vi "RMS Current Check.vi"(8 "error in":errorcluster, 10 "WaitMoniter Input":T4={"Wait Time(S)"=10.0, "Chamber Temp(Deg C)"=10.0, "Chamber Temp Tolerance(%)"=10.0, "RMS Current(A)"=10.0, "RMS Current Tolerance(%)"=10.0, "Temperature Control"=FALSE, "RMS Control"=FALSE, "RMS Current Min(A)"=10.0, "RMS Current Max(A)"=10.0, "Chamber Temp Min(Deg C)"=10.0, "Chamber Temp Max(Deg C)"=10.0, "HVPPS Current Max(A)"=10.0, "HVPPS Control"=FALSE, "HVPPS Current(A)"=10.0} {"HVPPS Current(A)" format="%#_13g"; "HVPPS Current Max(A)" format="%#_13g"; "Chamber Temp Max(Deg C)" format="%#_13g"; "Chamber Temp Min(Deg C)" format="%#_13g"; "RMS Current Max(A)" format="%#_13g"; "RMS Current Min(A)" format="%#_13g"; "RMS Current Tolerance(%)" format="%#_13g"; "RMS Current(A)" format="%#_13g"; "Chamber Temp Tolerance(%)" format="%#_13g"; "Chamber Temp(Deg C)" format="%#_13g"; "Wait Time(S)" format="%#_13g"}, 11 "Data Cluster":T1={"Chamber Address"={"Starting Address"=0, "Data Length"=0}, "Modbus RTU"={"unit ID"=1, "serial type"=enum."RTU", "baud rate"=9600, "parity (even)"=2, "flow control (none)"=0, "VISA resource name"=""}, "Temparature PASS?"=FALSE, "RMS Current PASS?"=FALSE, "Ping PASS?"=FALSE, "WaitMonitor_Class"=refnum, "Status Update"="", "Test Mode"=0, "Sequence Context"=refnum, "Running?"=FALSE, "RMS_FAIL_Count"=0, "Current Temperature"=0.0, "Target Temperature"=0.0, "RMS_Current"=[], "PowerStatus"={"Chamber IP Ping"=FALSE, "RAW_Power_Status"=FALSE, "PDU1_Status_Instrument_Rack"=FALSE, "PDU2_Status_PowerSupply_Rack_1"=FALSE, "PDU3_Status_PowerSupply_Rack_2"=FALSE}, "Monitor_Interval(S)"=0.0, "Current_Monitor_Interval(S)"=0.0, "RMS_Refresh?"=FALSE, "RTD Temperature(Deg C)"=0.0, "AbortTime(S)"=0.0, "HVPPS_Current"=[], "HVPPS Current PASS?"=FALSE} {"Modbus RTU"."parity (even)" items=["None", "Odd", "Even", "Mark", "Space"]; "Modbus RTU"."flow control (none)" items=["None", "XON/XOFF", "RTS/CTS", "XON/XOFF & RTS/CTS", "DTR/DSR", "XON/XOFF & DTR/DSR"]}) -> (0 "error out":errorcluster, 3 "Data Cluster out":T1={"Chamber Address"={"Starting Address"=0, "Data Length"=0}, "Modbus RTU"={"unit ID"=1, "serial type"=enum."RTU", "baud rate"=9600, "parity (even)"=2, "flow control (none)"=0, "VISA resource name"=""}, "Temparature PASS?"=FALSE, "RMS Current PASS?"=FALSE, "Ping PASS?"=FALSE, "WaitMonitor_Class"=refnum, "Status Update"="", "Test Mode"=0, "Sequence Context"=refnum, "Running?"=FALSE, "RMS_FAIL_Count"=0, "Current Temperature"=0.0, "Target Temperature"=0.0, "RMS_Current"=[], "PowerStatus"={"Chamber IP Ping"=FALSE, "RAW_Power_Status"=FALSE, "PDU1_Status_Instrument_Rack"=FALSE, "PDU2_Status_PowerSupply_Rack_1"=FALSE, "PDU3_Status_PowerSupply_Rack_2"=FALSE}, "Monitor_Interval(S)"=0.0, "Current_Monitor_Interval(S)"=0.0, "RMS_Refresh?"=FALSE, "RTD Temperature(Deg C)"=0.0, "AbortTime(S)"=0.0, "HVPPS_Current"=[], "HVPPS Current PASS?"=FALSE} {"Modbus RTU"."parity (even)" items=["None", "Odd", "Even", "Mark", "Space"]; "Modbus RTU"."flow control (none)" items=["None", "XON/XOFF", "RTS/CTS", "XON/XOFF & RTS/CTS", "DTR/DSR", "XON/XOFF & DTR/DSR"]})   [LabVIEW 2023, in "HardwareAbstractionLayer_LVOOP.lvlib" / "Wait Monitor.lvclass"]
uses:
  Wait Monitor.lvclass
  Teststand Steptypes/WaitMoniter/Control/Moniter Step Control.ctl
  Control/Data Cluster.ctl
  <vilib>/addons/TestStand/_TSLegacy.llb/LabVIEW Test - Sequence Context.ctl
  Teststand Steptypes/PowerMonitor/Control/PowerData.ctl
  Teststand Steptypes/CAN/STP/Steptypes/Control/STP Data.ctl
  CAN/CAN Application Protocols/STP Protocol_class/Ctrls/STP CMD.ctl
  Wait Monitor.lvclass/Wait Monitor.ctl
  Teststand/Teststand.lvclass
  CAN/CAN Application Protocols/STP Protocol_class/STP Protocol.lvclass
  Teststand Steptypes/LTT_TeststandSteptypes.lvlib
  <userlib>/_OpenG.lib/error/error.llb/openg_error.lvlib
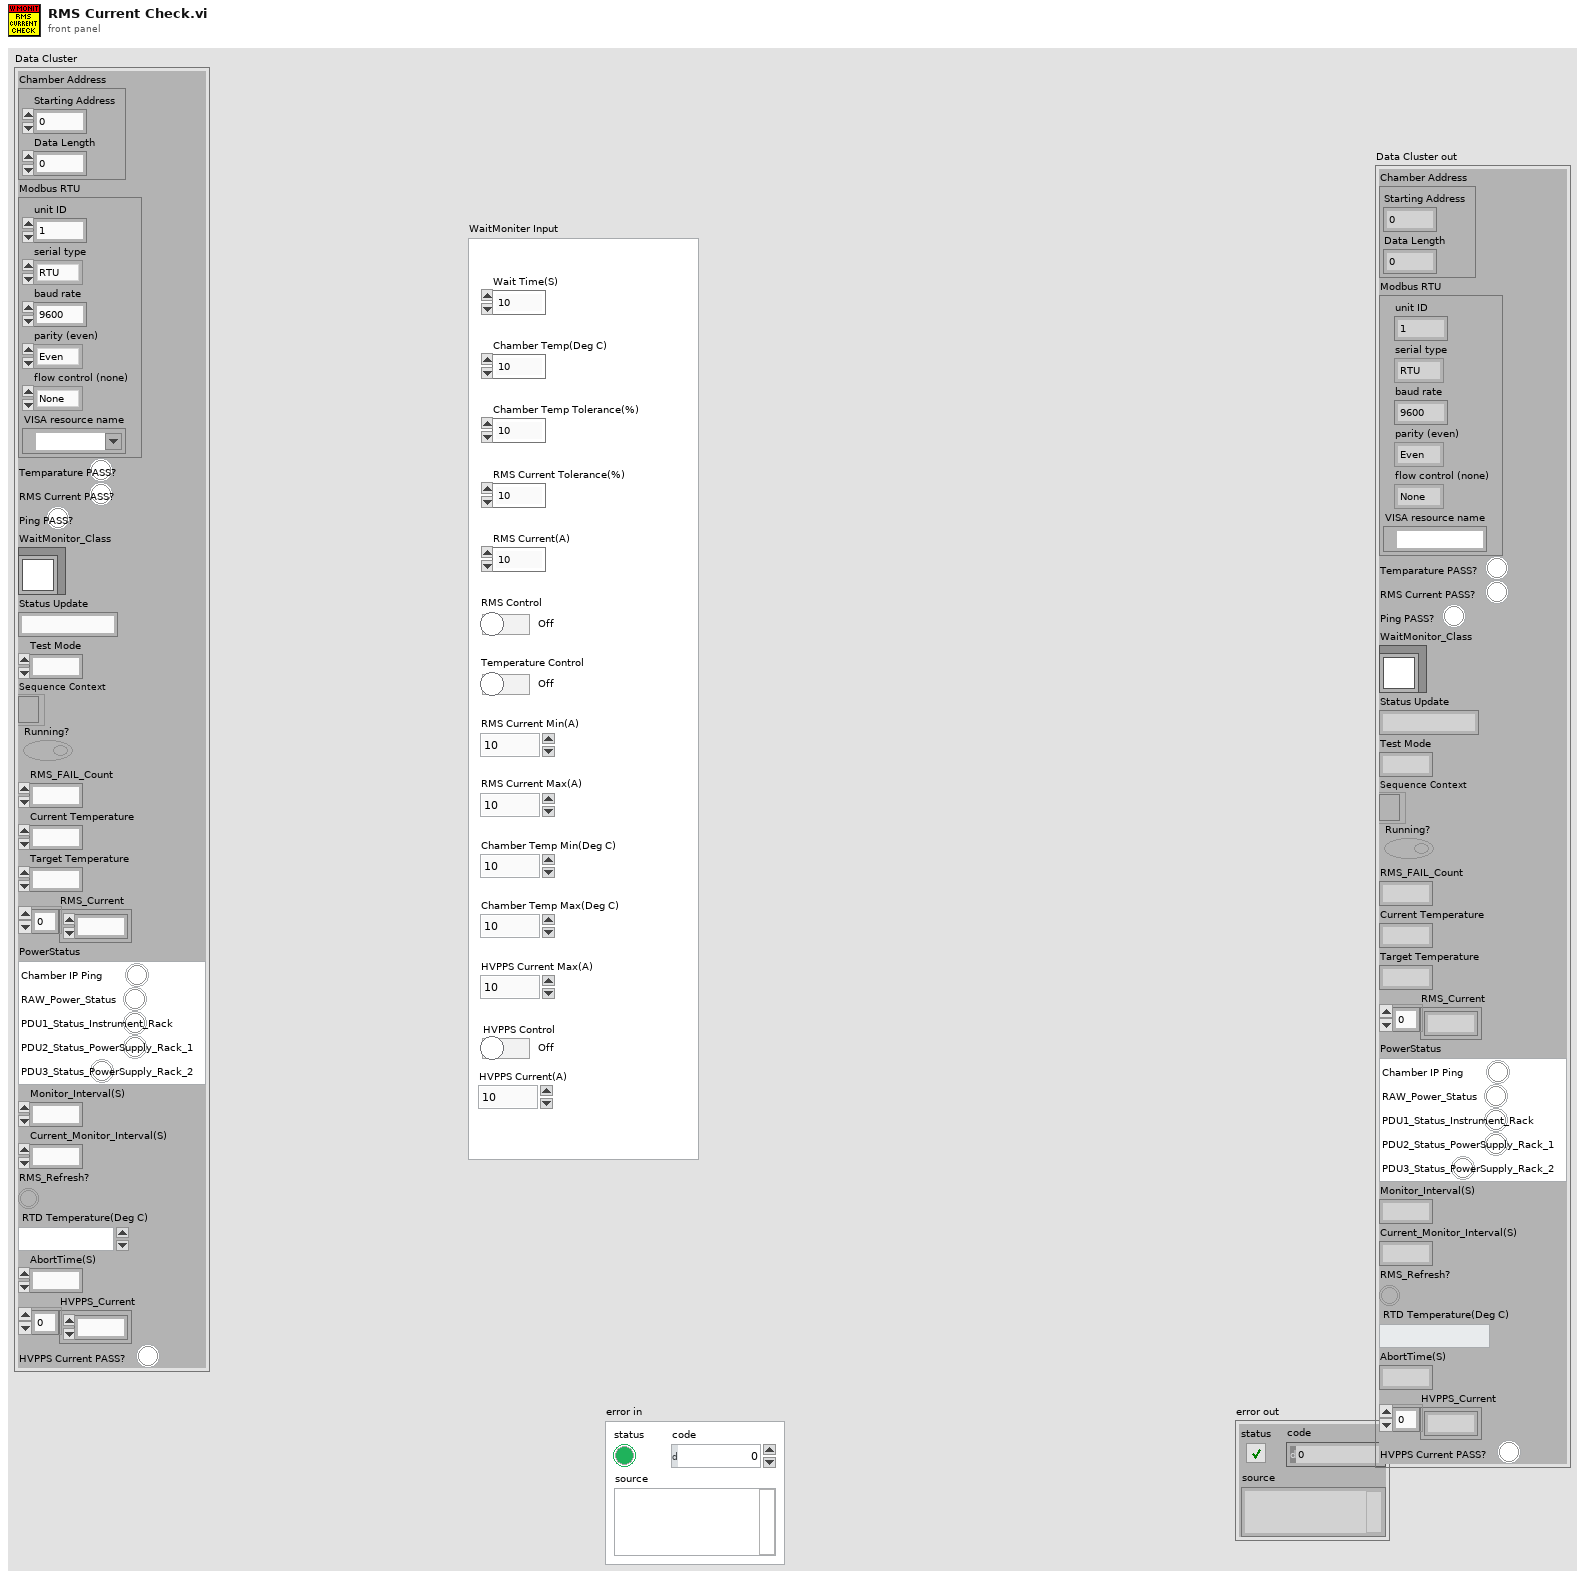
[diagram p1: front panel]
types:
  T1 = typedef "HardwareAbstractionLayer_LVOOP.lvlib/Wait Monitor.lvclass/Data Cluster.ctl" = cluster{"Chamber Address":cluster{"Starting Address":u16, "Data Length":u16}, "Modbus RTU":cluster{"unit ID":u8, "serial type":enum16{"RTU", "ASCII"}, "baud rate":u32, "parity (even)":u16, "flow control (none)":u16, "VISA resource name":refnum<visa-resource-name>}, "Temparature PASS?":bool, "RMS Current PASS?":bool, "Ping PASS?":bool, "WaitMonitor_Class":refnum<class "Wait Monitor.lvclass">, "Status Update":string, "Test Mode":u16, "Sequence Context":T2, "Running?":bool, "RMS_FAIL_Count":u16, "Current Temperature":dbl, "Target Temperature":dbl, "RMS_Current":dbl[], "PowerStatus":T3, "Monitor_Interval(S)":dbl, "Current_Monitor_Interval(S)":dbl, "RMS_Refresh?":bool, "RTD Temperature(Deg C)":dbl, "AbortTime(S)":dbl, "HVPPS_Current":dbl[], "HVPPS Current PASS?":bool}
  T2 = typedef "LabVIEW Test - Sequence Context.ctl" = refnum<k7>
  T3 = typedef "LTT_TeststandSteptypes.lvlib/PowerData.ctl" = cluster{"Chamber IP Ping":bool, "RAW_Power_Status":bool, "PDU1_Status_Instrument_Rack":bool, "PDU2_Status_PowerSupply_Rack_1":bool, "PDU3_Status_PowerSupply_Rack_2":bool}
  T4 = typedef "HardwareAbstractionLayer_LVOOP.lvlib/Wait Monitor.lvclass/Moniter Step Control.ctl" = cluster{"Wait Time(S)":dbl, "Chamber Temp(Deg C)":dbl, "Chamber Temp Tolerance(%)":dbl, "RMS Current(A)":dbl, "RMS Current Tolerance(%)":dbl, "Temperature Control":bool, "RMS Control":bool, "RMS Current Min(A)":dbl, "RMS Current Max(A)":dbl, "Chamber Temp Min(Deg C)":dbl, "Chamber Temp Max(Deg C)":dbl, "HVPPS Current Max(A)":dbl, "HVPPS Control":bool, "HVPPS Current(A)":dbl}
  T5 = typedef "LTT_TeststandSteptypes.lvlib/STP Data.ctl" = cluster{"ECU CAN Port":string, "CMD":T6, "CAN Write Data":u8[], "Response Decoder":enum16{"String", "Number", "Boolean"}, "String":cluster{"Start Index":i32, "Length":i32}, "Number":cluster{"MSB Index":i32, "LSB Index":i32}, "Boolean":cluster{"Index":i32, "Bool":cluster{"7":bool, "6":bool, "5":bool, "4":bool, "3":bool, "2":bool, "1":bool, "0":bool, "7 Enabled":bool, "6 Enabled":bool, "5 Enabled":bool, "4 Enabled":bool, "3 Enabled":bool, "2 Enabled":bool, "1 Enabled":bool, "0 Enabled":bool}}}
  T6 = typedef "HardwareAbstractionLayer_LVOOP.lvlib/CAN Application Protocols Lib.lvlib/STP Protocol.lvclass/STP CMD.ctl" = u8
  T7 = typedef "HardwareAbstractionLayer_LVOOP.lvlib/Teststand.lvclass/Teststand Status Control.ctl" = cluster{"Terminating or Aborting":bool, "Stop":bool, "Socket Count":i16, "Selected Sockets":i16[]}
  T8 = typedef "LTT_TeststandSteptypes.lvlib/STP Out Data.ctl" = cluster{"String Data":string, "Numeric Data":dbl, "Boolean Data":bool, "RequestTimeout?":bool, "ResponseData":u8[], "PositiveResponse?":bool}
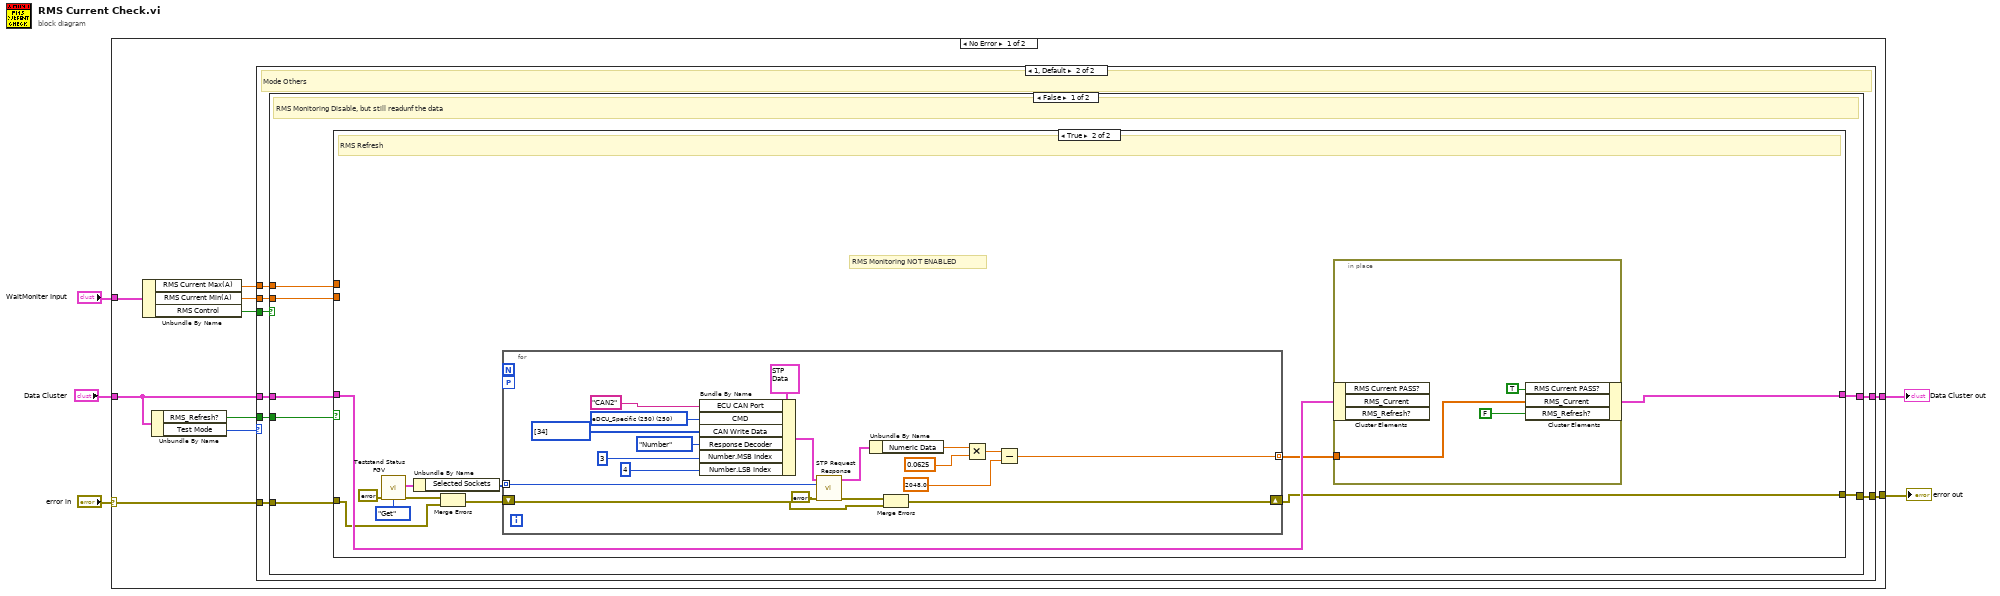
[diagram p0: block diagram]
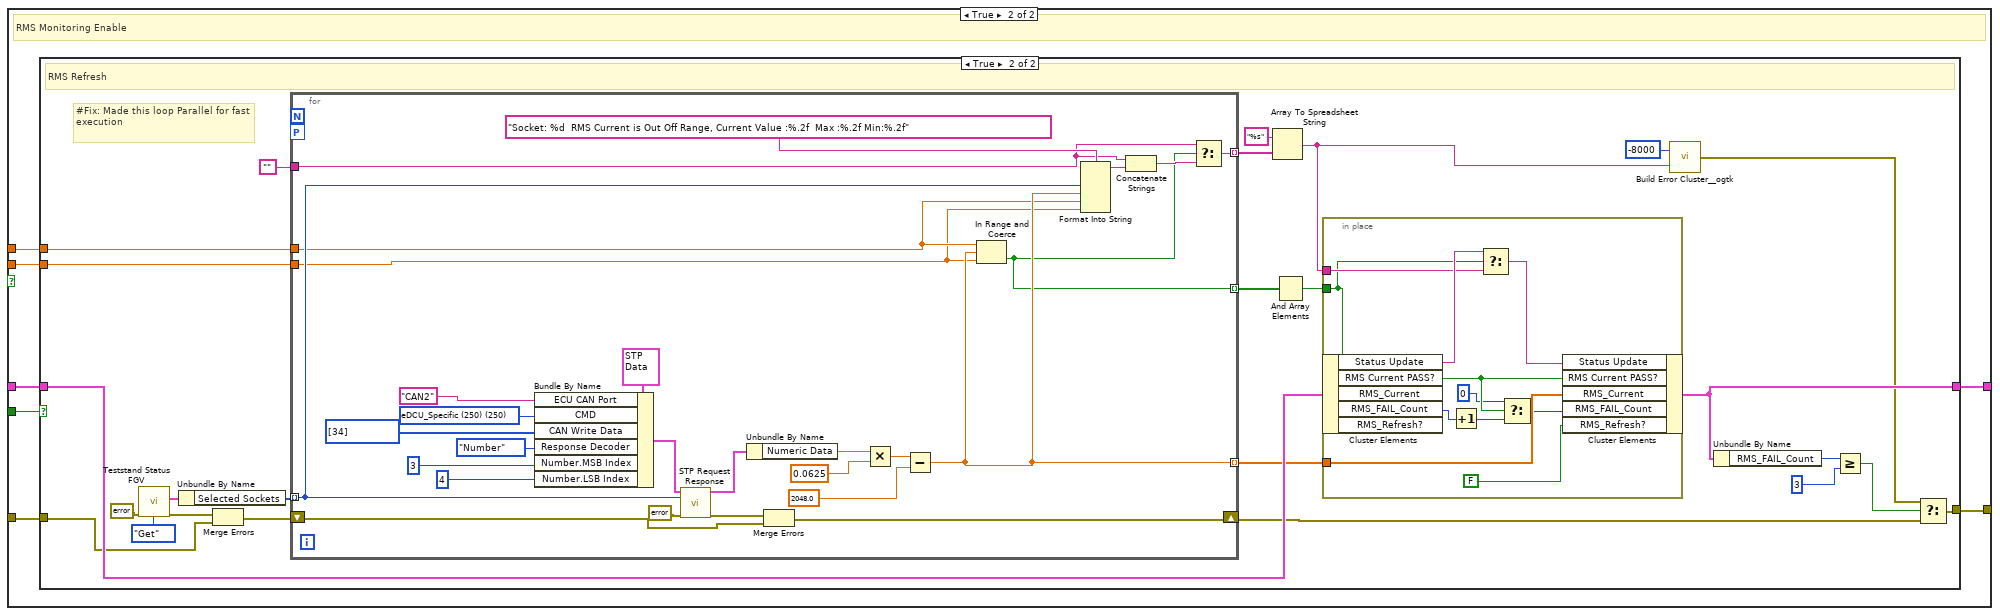
[diagram p4: hidden frame]
diagram:
  n1 = case shown="No Error" "error in" {
    selector: "error in" -> [w15 w140]
    tunnel: [w14 w140] -> w4
    tunnel: "WaitMoniter Input" -> [w12 _]
    tunnel: "Data Cluster" -> [w10 w139]
    tunnel: [w11 w139] -> w1
    frame No Error {
      n2 = Unbundle By Name(w12) -> ("RMS Current Max(A)"=w8:dbl, "RMS Current Min(A)"=w7:dbl, "RMS Control"=w13:bool)
      n3 = Unbundle By Name(w10) -> ("RMS_Refresh?"=w9:bool, "Test Mode"=w6:u16)
      n4 = case shown="1, Default" w6 {
        tunnel: w15 -> [w17 w25]
        tunnel: [w17 w24] -> w14
        tunnel: w13 -> [_ w23]
        tunnel: [w16 w22] -> w11
        tunnel: w10 -> [w16 w21]
        tunnel: w9 -> [_ w20]
        tunnel: w8 -> [_ w19]
        tunnel: w7 -> [_ w18]
        frame 0 {
          # "Mode 0"
        }
        frame 1, Default {
          # "Mode Others"
          n5 = case shown="False" w23 {
            tunnel: w25 -> [w28 w74]
            tunnel: [w27 w71] -> w24
            tunnel: w21 -> [w31 w73]
            tunnel: [w26 w72] -> w22
            tunnel: w20 -> [w32 w70]
            tunnel: w19 -> [w29 w69]
            tunnel: w18 -> [w30 w68]
            frame False {
              # "RMS Monitoring NOT ENABLED"
              # "RMS Monitoring Disable, but still readunf the data"
              n6 = case shown="True" w32 {
                tunnel: w28 -> [w34 w36]
                tunnel: w31 -> [w33 w41]
                tunnel: [w33 w39] -> w26
                tunnel: [w34 w35] -> w27
                tunnel: w29 -> [_ _]
                tunnel: w30 -> [_ _]
                frame False {
                  # "RMS Refresh NOT True"
                  # "RMS RefreshOff"
                }
                frame True {
                  # "RMS Refresh"
                  n7 = call "Teststand Status FGV.vi"("error in"=errorcluster {"status"=FALSE, "code"=0, "source"=""}, "Option"=enum16{"Set", "Get"}."Get") -> ("error out"=w42:errorcluster, "Teststand Status Out"=w44:T7)  [unwired: 8 in]
                  n8 = Unbundle By Name(w44) -> ("Selected Sockets"=w43:i16[])
                  n9 = Merge Errors(w42, w36) -> (w37:errorcluster)
                  n10 = for {
                    tunnel: w43 -> [w49] mode=indexing
                    shift-right: [w50] -> w35
                    shift-left: w37 -> [w67]
                    tunnel: [w51] -> w40 mode=indexing
                    workers-P: _ -> [_]
                    w60 = T6 250 items=["TSW_VERSION(130)"=130, "WAIT_EVENT(132)"=132, "SEQUENCER(133)"=133, "TSW_RESET(150)"=150, "CONFIG_ECU(151)"=151, "TEST_CORE (152)"=152, "TEST_WATCHDOG (153)"=153, "TEST_MONITORING (154)"=154, "READ_MEMORY (162)"=162, "WRITE_ERASE_MEMORY (164)"=164, "COMM_EXTERNAL (190)"=190, "COMM_INTERNAL (195)"=195, "GET_ANALOG_INPUT (210)"=210, "GET_DIGITAL_INPUT (211)"=211, "GET_FREQUENCY_INPUT (212)"=212, "TEST_INPUT_STRUCTURE (214)"=214, "GENERATE_OUTPUT_SIGNAL (220)"=220, "GENERATE_SYNCHRONIZED_OUTPUT_SIGNALS (221)"=221, "eDCU_Specific (250)"=250] ("CMD")
                    n11 = Bundle By Name(cluster=T5 {"ECU CAN Port"="CAN2", "CMD"=250, "CAN Write Data"=[34], "Response Decoder"=enum."String", "String"={"Start Index"=0, "Length"=-1}, "Number"={"MSB Index"=0, "LSB Index"=1}, "Boolean"={"Index"=0, "Bool"={"7"=FALSE, "6"=FALSE, "5"=FALSE, "4"=FALSE, "3"=FALSE, "2"=FALSE, "1"=FALSE, "0"=FALSE, "7 Enabled"=FALSE, "6 Enabled"=FALSE, "5 Enabled"=FALSE, "4 Enabled"=FALSE, "3 Enabled"=FALSE, "2 Enabled"=FALSE, "1 Enabled"=FALSE, "0 Enabled"=FALSE}}} ("STP Data in"), "ECU CAN Port"="CAN2", "CMD"=w60, "CAN Write Data"=u8[] [34], "Response Decoder"=enum16{"String", "Number", "Boolean"}."Number", "Number.MSB Index"=3, "Number.LSB Index"=4) -> (w52:T5)
                    n12 = call "STP Request Response.vi"("error in"=errorcluster {"status"=FALSE, "code"=0, "source"=""}, "Socket No"=w49, "STP Data in"=w52) -> ("error out"=w66:errorcluster, "STP Data Out"=w65:T8)  [unwired: 5 in, 2 out]
                    n13 = Unbundle By Name(w65) -> ("Numeric Data"=w53:dbl)
                    n14 = Merge Errors(w66, w67) -> (w50:errorcluster)
                    n15 = Multiply(x=w53, y=0.0625) -> (x*y=w63:dbl)
                    n16 = Subtract(x=w63, y=2048.0) -> (x-y=w51:dbl)
                  }
                  n17 = in-place {
                    in-place-border: w40 -> [w48]
                    n18 = in-place-cluster #1(w41) -> ()  [unwired: 3 out]
                    n19 = in-place-cluster #1("RMS Current PASS?"=TRUE, "RMS_Current"=w48, "RMS_Refresh?"=FALSE) -> (w39:T1)
                  }
                }
              }
            }
            frame True {
              # "RMS Monitoring Enable"
              n20 = case shown="True" w70 {
                tunnel: w74 -> [w76 w80]
                tunnel: w73 -> [w75 w96]
                tunnel: [w75 w92] -> w72
                tunnel: [w76 w84] -> w71
                tunnel: w69 -> [_ w86]
                tunnel: w68 -> [_ w85]
                frame False {
                  # "RMS Refresh NOT True"
                  # "RMS Refresh Off"
                }
                frame True {
                  # "#Fix: Made this loop Parallel for fast execution"
                  # "RMS Refresh"
                  n21 = call "Teststand Status FGV.vi"("error in"=errorcluster {"status"=FALSE, "code"=0, "source"=""}, "Option"=enum16{"Set", "Get"}."Get") -> ("error out"=w98:errorcluster, "Teststand Status Out"=w100:T7)  [unwired: 8 in]
                  n22 = Unbundle By Name(w100) -> ("Selected Sockets"=w99:i16[])
                  n23 = Merge Errors(w98, w80) -> (w81:errorcluster)
                  n24 = for {
                    tunnel: w99 -> [w115] mode=indexing
                    shift-right: [w116] -> w88
                    shift-left: w81 -> [w138]
                    tunnel: [w112] -> w97 mode=indexing
                    tunnel: [w121] -> w94 mode=indexing
                    tunnel: w86 -> [w114]
                    tunnel: w85 -> [w113]
                    workers-P: _ -> [_]
                    tunnel: "" -> [w117]
                    tunnel: [w119] -> w79 mode=indexing
                    w131 = T6 250 items=["TSW_VERSION(130)"=130, "WAIT_EVENT(132)"=132, "SEQUENCER(133)"=133, "TSW_RESET(150)"=150, "CONFIG_ECU(151)"=151, "TEST_CORE (152)"=152, "TEST_WATCHDOG (153)"=153, "TEST_MONITORING (154)"=154, "READ_MEMORY (162)"=162, "WRITE_ERASE_MEMORY (164)"=164, "COMM_EXTERNAL (190)"=190, "COMM_INTERNAL (195)"=195, "GET_ANALOG_INPUT (210)"=210, "GET_DIGITAL_INPUT (211)"=211, "GET_FREQUENCY_INPUT (212)"=212, "TEST_INPUT_STRUCTURE (214)"=214, "GENERATE_OUTPUT_SIGNAL (220)"=220, "GENERATE_SYNCHRONIZED_OUTPUT_SIGNALS (221)"=221, "eDCU_Specific (250)"=250] ("CMD")
                    n25 = Bundle By Name(cluster=T5 {"ECU CAN Port"="CAN2", "CMD"=250, "CAN Write Data"=[34], "Response Decoder"=enum."String", "String"={"Start Index"=0, "Length"=-1}, "Number"={"MSB Index"=0, "LSB Index"=1}, "Boolean"={"Index"=0, "Bool"={"7"=FALSE, "6"=FALSE, "5"=FALSE, "4"=FALSE, "3"=FALSE, "2"=FALSE, "1"=FALSE, "0"=FALSE, "7 Enabled"=FALSE, "6 Enabled"=FALSE, "5 Enabled"=FALSE, "4 Enabled"=FALSE, "3 Enabled"=FALSE, "2 Enabled"=FALSE, "1 Enabled"=FALSE, "0 Enabled"=FALSE}}} ("STP Data in"), "ECU CAN Port"="CAN2", "CMD"=w131, "CAN Write Data"=u8[] [34], "Response Decoder"=enum16{"String", "Number", "Boolean"}."Number", "Number.MSB Index"=3, "Number.LSB Index"=4) -> (w123:T5)
                    n26 = call "STP Request Response.vi"("error in"=errorcluster {"status"=FALSE, "code"=0, "source"=""}, "Socket No"=w115, "STP Data in"=w123) -> ("error out"=w137:errorcluster, "STP Data Out"=w136:T8)  [unwired: 5 in, 2 out]
                    n27 = Unbundle By Name(w136) -> ("Numeric Data"=w124:dbl)
                    n28 = Merge Errors(w137, w138) -> (w116:errorcluster)
                    n29 = Multiply(x=w124, y=0.0625) -> (x*y=w134:dbl)
                    n30 = Subtract(x=w134, y=2048.0) -> (x-y=w121:dbl)
                    n31 = In Range and Coerce(upper limit=w114, x=w121, lower limit=w113) -> (In Range?=w112:bool)  [unwired: 1 out]
                    n32 = Format Into String(format string="Socket: %d  RMS Current is Out Off Range, Current Value :%.2f  Max :%.2f Min:%.2f", w115, w121, w114, w113) -> (resulting string=w120:string)  [unwired: 2 in, 1 out]
                    n33 = Concatenate Strings(w117, w120) -> (w118:string)
                    n34 = Select(t=w117, s=w112, f=w118) -> (s? t:f=w119:string)
                  }
                  n35 = Array To Spreadsheet String(array=w79, 3:"%s" ("format string")) -> (spreadsheet string=w78:string)  [unwired: 1 in]
                  n36 = And Array Elements(Boolean array=w97) -> (logical AND=w95:bool)
                  n37 = in-place {
                    in-place-border: w95 -> [w107]
                    in-place-border: w94 -> [w111]
                    in-place-border: w78 -> [w109]
                    n38 = in-place-cluster #2(w96) -> ("Status Update"=w110:string, "RMS_FAIL_Count"=w104:u16)  [unwired: 3 out]
                    n39 = Increment(x=w104) -> (x+1=w105:u16)
                    n40 = Select(t=w110, s=w107, f=w109) -> (s? t:f=w108:string)
                    n41 = Select(t=u16 0, s=w107, f=w105) -> (s? t:f=w106:u16)
                    n42 = in-place-cluster #2("Status Update"=w108, "RMS Current PASS?"=w107, "RMS_Current"=w111, "RMS_FAIL_Count"=w106, "RMS_Refresh?"=FALSE) -> (w92:T1)
                  }
                  n43 = call <userlib>:"Build Error Cluster__ogtk.vi"("String to Prepend to source (\"\")"=w78, "code"=-8000) -> ("error out"=w83:errorcluster)
                  n44 = Unbundle By Name(w92) -> ("RMS_FAIL_Count"=w91:u16)
                  n45 = Greater Or Equal?(x=w91, y=u16 3) -> (x >= y?=w89:bool)
                  n46 = Select(t=w83, s=w89, f=w88) -> (s? t:f=w84:errorcluster)
                }
              }
            }
          }
        }
      }
    }
    frame Error {
    }
  }
  "error out" <- w4
  "Data Cluster out" <- w1
